vi "display_1s_stim_9s_ISI_CS1_CS2_blocks.vi"() -> ()   [LabVIEW 2019]
uses:
  <vilib>/Analysis/Matrix/Datatypes/RealMatrix.ctl
  <vilib>/Utility/file.llb/Write Delimited Spreadsheet (DBL).vi
  <vilib>/Analysis/Matrix/NI_Matrix.lvlib
panel:
  out "Active trial":bool=TRUE
  out "ISI Time":dbl
  out "Stim TS":dbl
  out "Output":dbl[][](array[numeric])
  out "Output frame":T1
  out "Frame_clock":u32
  out "Array temp1":T1
  out "Elapsed Time":dbl
  out "Display":bool=TRUE
  out "Trial":u32=1
  out "reward":dbl[](array[numeric])
  out "stim_id":dbl[](array[numeric])
  out "stim_loaded":dbl
  out "Timings":dbl[](array[numeric])
  out "Stimuli Loaded?":bool
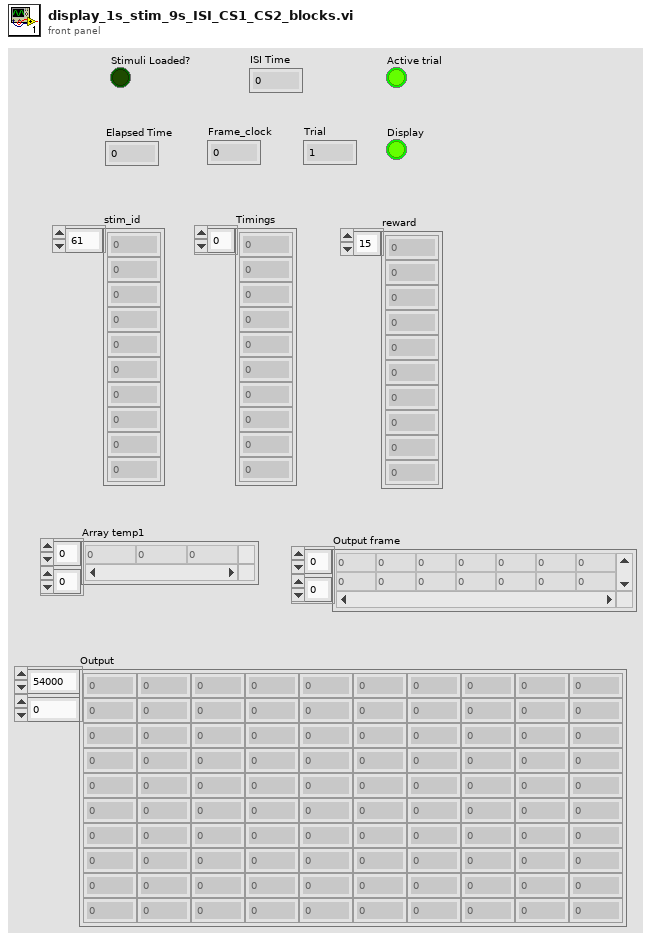
[diagram p1: front panel]
types:
  T1 = typedef "NI_Matrix.lvlib/RealMatrix.ctl" = dbl[][]
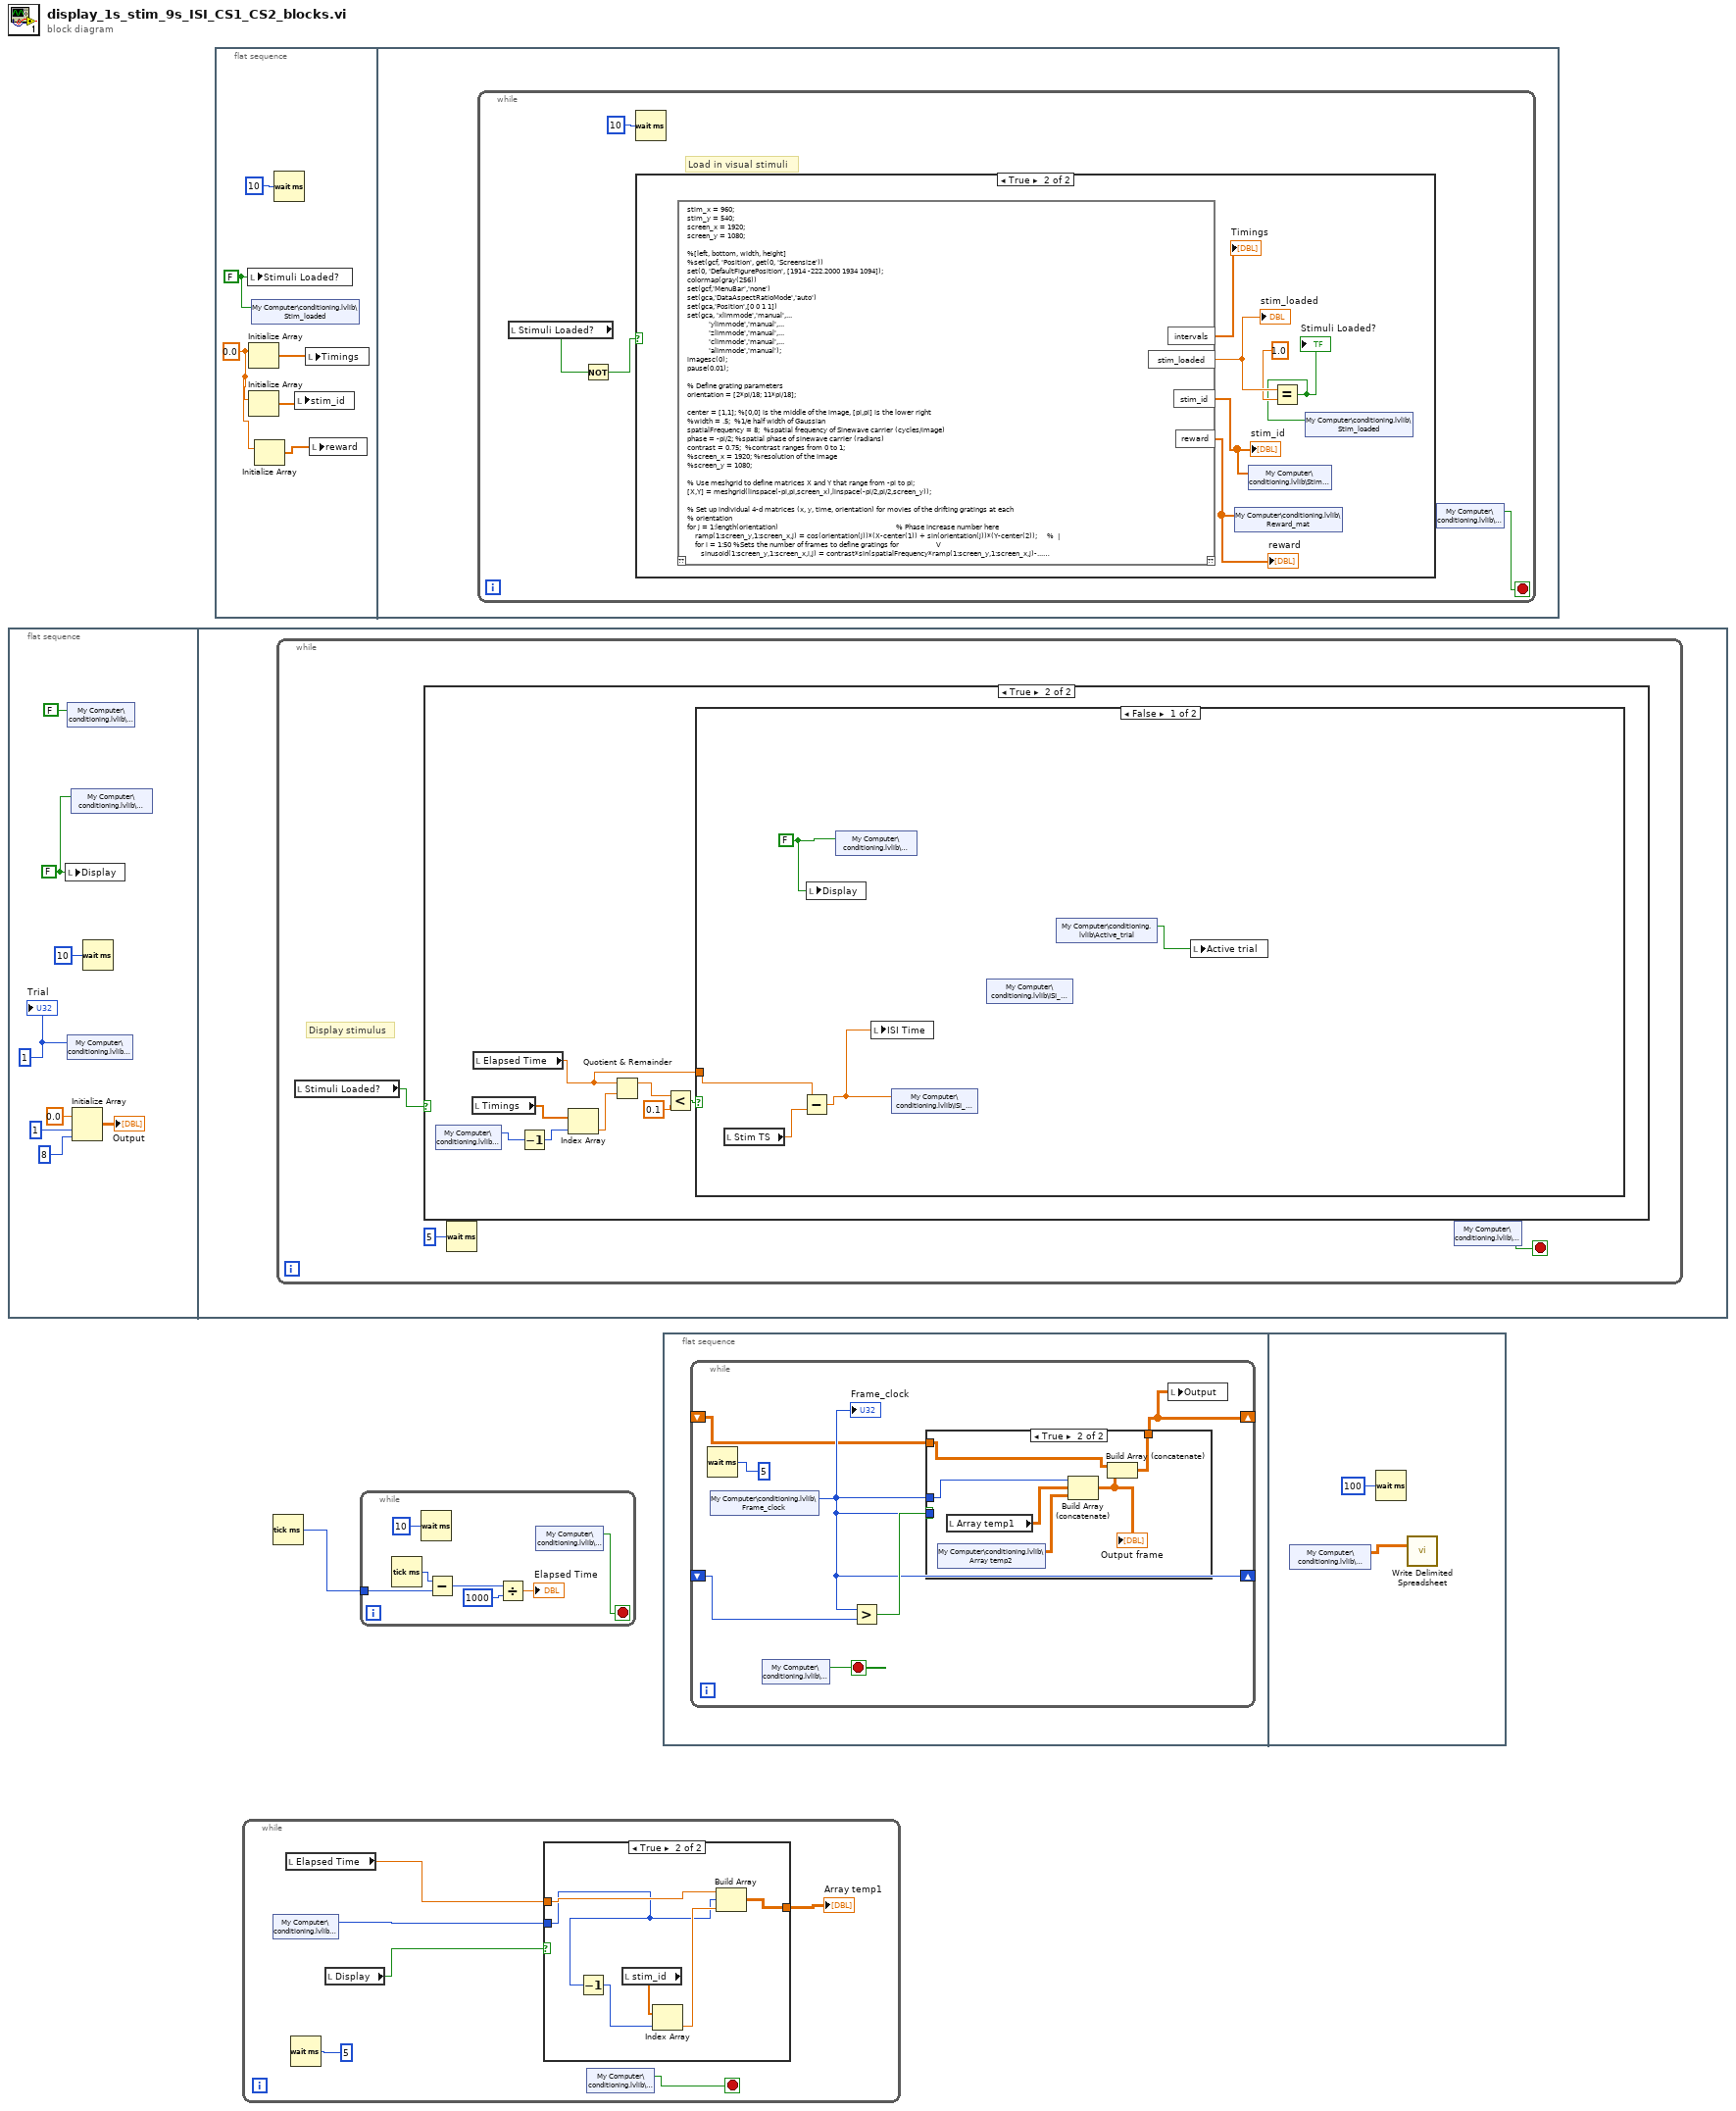
[diagram p0: block diagram]
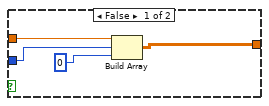
[diagram p2: hidden frame]
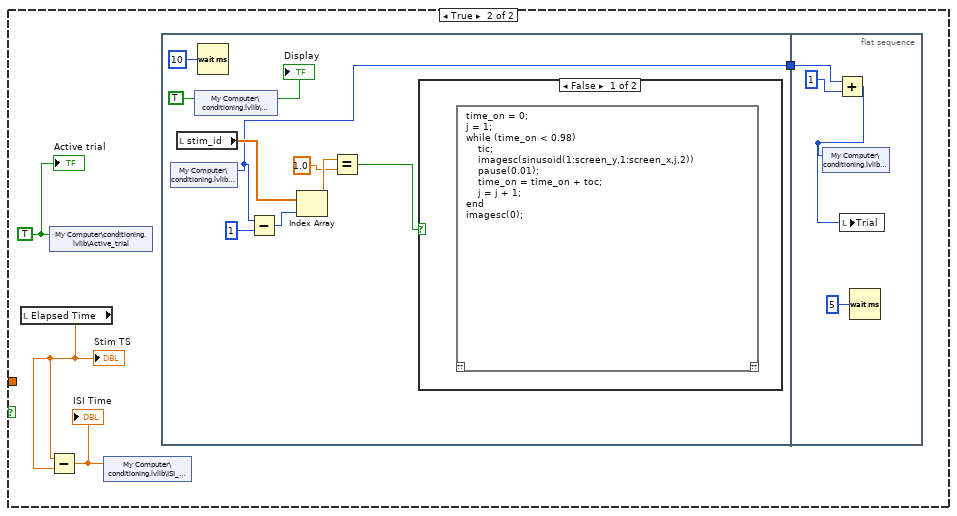
[diagram p6: hidden frame]
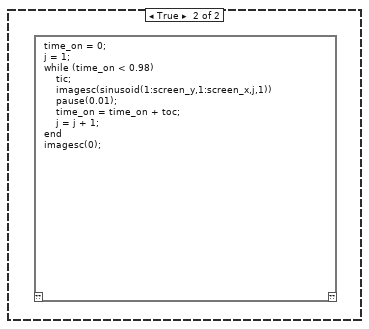
[diagram p7: hidden frame]
diagram:
  n1 = flat-sequence {
    frame #0 {
      w7 = FALSE ("Display")
      w9 = u32 1 ("Trial")
      n2 = local write "Display"(w7) -> ()
      n3 = shared-variable "My Computer\\conditioning.lvlib\\Stop"(FALSE ("Stop")) -> ()  [unwired: 1 in, 1 out]
      n4 = shared-variable "My Computer\\conditioning.lvlib\\Trial"(w9) -> ()  [unwired: 1 in, 1 out]
      n5 = shared-variable "My Computer\\conditioning.lvlib\\Display"(w7) -> ()  [unwired: 1 in, 1 out]
      n6 = Initialize Array(0.0 ("element"), 1 ("dimension size"), 8 ("dimension size")) -> (→"Output":dbl[][])
      n7 = Wait (ms)(milliseconds to wait=u32 10) -> ()  [unwired: 1 out]
      "Trial" <- w9
    }
    frame #1 {
      n8 = while {
        stop <- w11 stop-if-true
        # "Display stimulus"
        n9 = local read "Stimuli Loaded?"() -> (w10:bool)
        n10 = case shown="True" w10 {
          frame False {
          }
          frame True {
            n11 = shared-variable "My Computer\\conditioning.lvlib\\Trial"() -> (w16:u32)  [unwired: 1 in, 1 out]
            n12 = local read "Timings"() -> (w17:dbl[])
            n13 = local read "Elapsed Time"() -> (w13:dbl)
            n14 = Decrement(x=w16) -> (x-1=w15:u32)
            n15 = Index Array(array=w17, index=w15) -> (element=w14:dbl)
            n16 = Quotient & Remainder(x=w13, y=w14) -> (x-y*floor(x/y)=w20:dbl)  [unwired: 1 out]
            n17 = Less?(x=w20, y=0.1) -> (x < y?=w18:bool)
            n18 = case shown="False" w18 {
              tunnel: w13 -> [w24 _]
              frame False {
                w25 = FALSE ("Display")
                n19 = local read "Stim TS"() -> (w23:dbl)
                n20 = Subtract(x=w24, y=w23) -> (x-y=w22:dbl)
                n21 = local write "Display"(w25) -> ()
                n22 = shared-variable "My Computer\\conditioning.lvlib\\Display"(w25) -> ()  [unwired: 1 in, 1 out]
                n23 = local write "ISI Time"(w22) -> ()
                n24 = shared-variable "My Computer\\conditioning.lvlib\\ISI_Time"(w22) -> ()  [unwired: 1 in, 1 out]
                n25 = shared-variable "My Computer\\conditioning.lvlib\\ISI_Time"() -> ()  [unwired: 1 in, 2 out]
                n26 = shared-variable "My Computer\\conditioning.lvlib\\Active_trial"() -> (w21:bool)  [unwired: 1 in, 1 out]
                n27 = local write "Active trial"(w21) -> ()
              }
              frame True {
                w27 = TRUE ("Active_trial")
                n28 = local read "Elapsed Time"() -> (w28:dbl)
                "Stim TS" <- w28
                n29 = Subtract(x=w28, y=w28) -> (x-y=w26:dbl)
                "ISI Time" <- w26
                n30 = shared-variable "My Computer\\conditioning.lvlib\\Active_trial"(w27) -> ()  [unwired: 1 in, 1 out]
                n31 = shared-variable "My Computer\\conditioning.lvlib\\ISI_Time"(w26) -> ()  [unwired: 1 in, 1 out]
                n32 = flat-sequence {
                  tunnel: [w32] -> w29
                  tunnel: w29 -> [w42]
                  frame #0 {
                    w34 = TRUE ("Boolean")
                    n33 = shared-variable "My Computer\\conditioning.lvlib\\Trial"() -> (w32:u32)  [unwired: 1 in, 1 out]
                    n34 = local read "stim_id"() -> (w37:dbl[])
                    n35 = shared-variable "My Computer\\conditioning.lvlib\\Display"(w34) -> ()  [unwired: 1 in, 1 out]
                    n36 = Wait (ms)(milliseconds to wait=u32 10) -> ()  [unwired: 1 out]
                    n37 = Subtract(x=w32, y=u32 1) -> (x-y=w33:u32)
                    n38 = Index Array(array=w37, index=w33) -> (element=w36:dbl)
                    n39 = Equal?(x=w36, y=1.0) -> (x = y?=w30:bool)
                    n40 = case shown="False" w30 {
                      frame False {
                        n41 = script code="time_on = 0;\nj = 1;\nwhile (time_on < 0.98)\n    tic;\n    imagesc(sinusoid(1:screen_y,1:screen_x,j,2))\n    pause(0.01);\n    time_on = time_on + toc;\n    j = j + 1;\nend\nimagesc(0);"() -> ()  [unwired: 1 in, 1 out]
                      }
                      frame True {
                        n42 = script code="time_on = 0;\nj = 1;\nwhile (time_on < 0.98)\n    tic;\n    imagesc(sinusoid(1:screen_y,1:screen_x,j,1))\n    pause(0.01);\n    time_on = time_on + toc;\n    j = j + 1;\nend\nimagesc(0);"() -> ()  [unwired: 1 in, 1 out]
                      }
                    }
                    "Display" <- w34
                  }
                  frame #1 {
                    n43 = Add(x=w42, y=u32 1) -> (x+y=w40:u32)
                    n44 = shared-variable "My Computer\\conditioning.lvlib\\Trial"(w40) -> ()  [unwired: 1 in, 1 out]
                    n45 = local write "Trial"(w40) -> ()
                    n46 = Wait (ms)(milliseconds to wait=u32 5) -> ()  [unwired: 1 out]
                  }
                }
                "Active trial" <- w27
              }
            }
          }
        }
        n47 = Wait (ms)(milliseconds to wait=u32 5) -> ()  [unwired: 1 out]
        n48 = shared-variable "My Computer\\conditioning.lvlib\\Stop"() -> (w11:bool)  [unwired: 1 in, 1 out]
      }
    }
  }
  n49 = flat-sequence {
    frame #0 {
      w45 = 0.0 ("element")
      w43 = FALSE ("Stimuli Loaded?")
      n50 = local write "Stimuli Loaded?"(w43) -> ()
      n51 = Initialize Array(w45) -> (w47:dbl[])  [unwired: 1 in]
      n52 = Initialize Array(w45) -> (w46:dbl[])  [unwired: 1 in]
      n53 = shared-variable "My Computer\\conditioning.lvlib\\Stim_loaded"(w43) -> ()  [unwired: 1 in, 1 out]
      n54 = Initialize Array(w45) -> (w44:dbl[])  [unwired: 1 in]
      n55 = Wait (ms)(milliseconds to wait=u32 10) -> ()  [unwired: 1 out]
      n56 = local write "stim_id"(w46) -> ()
      n57 = local write "Timings"(w47) -> ()
      n58 = local write "reward"(w44) -> ()
    }
    frame #1 {
      n59 = while {
        stop <- w51 stop-if-true
        # "Load in visual stimuli"
        n60 = local read "Stimuli Loaded?"() -> (w50:bool)
        n61 = Not(x=w50) -> (.not. x?=w49:bool)
        n62 = Wait (ms)(milliseconds to wait=u32 10) -> ()  [unwired: 1 out]
        n63 = case shown="True" w49 {
          frame False {
          }
          frame True {
            n64 = script code="stim_x = 960;\nstim_y = 540;\nscreen_x = 1920;\nscreen_y = 1080;\n\n%[left, bottom, width, height]\n%set(gcf, 'Position', get(0, 'Screensize'))\nset(0, 'DefaultFigurePosition', [1914 -222.2000 1934 1094]);\ncolormap(gray(256))\nset(gcf,'MenuBar','none')\nset(gca,'DataAspectRatioMode','auto')\nset(gca,'Position',[0 0 1 1])\nset(gca, 'xlimmode','manual',...\n           'ylimmode','manual',...\n           'zlimmode','manual',...\n           'climmode','manual',...\n           'alimmode','manual');\nimagesc(0);\npause(0.01);\n\n% Define grating parameters\norientation = [2*pi/18; 11*pi/18];\n\ncenter = [1,1]; %[0,0] is the middle of the image, [pi,pi] is the lower right\n%width = .5;  %1/e half width of Gaussian\nspatialFrequency = 8;  %spatial frequency of Sinewave carrier (cycles/image)\nphase = -pi/2; %spatial phase of sinewave carrier (radians)\ncontrast = 0.75;  %contrast ranges from 0 to 1;\n%screen_x = 1920; %resolution of the image  \n%screen_y = 1080;\n\n% Use meshgrid to define matrices X and Y that range from -pi to pi;\n[X,Y] = meshgrid(linspace(-pi,pi,screen_x),linspace(-pi/2,pi/2,screen_y));\n\n% Set up individual 4-d matrices (x, y, time, orientation) for movies of the drifting gratings at each\n% orientation\nfor j = 1:length(orientation)                                                            % Phase increase number here\n    ramp(1:screen_y,1:screen_x,j) = cos(orientation(j))*(X-center(1)) + sin(orientation(j))*(Y-center(2));     %  |\n    for i = 1:50 %Sets the number of frames to define gratings for                   V\n       sinusoid(1:screen_y,1:screen_x,i,j) = contrast*sin(spatialFrequency*ramp(1:screen_y,1:screen_x,j)-...\n           (phase+(2*pi*(i-1)*(-30)/360))); %Number before '/360' sets the phase increase\n    end\nend\n\nintervals = [ones(1,204)*12];\nstim_id = [ones(1,34)*1 ones(1,34)*2 ones(1,34)*1 ones(1,34)*2 ones(1,34)*1 ones(1,34)*2];\nreward = [ones(1,204)];\n\nstim_loaded = 1;" ("Script Node")() -> ("stim_loaded"=w58:dbl, "intervals"=→"Timings":dbl[], "stim_id"=w53:dbl[], "reward"=w55:dbl[])  [unwired: 1 in, 1 out]
            "stim_loaded" <- w58
            "stim_id" <- w53
            "reward" <- w55
            n65 = shared-variable "My Computer\\conditioning.lvlib\\Reward_mat"(w55) -> ()  [unwired: 1 in, 1 out]
            n66 = shared-variable "My Computer\\conditioning.lvlib\\Stim_ID"(w53) -> ()  [unwired: 1 in, 1 out]
            n67 = Equal?(x=w58, y=1.0) -> (x = y?=w54:bool)
            "Stimuli Loaded?" <- w54
            n68 = shared-variable "My Computer\\conditioning.lvlib\\Stim_loaded"(w54) -> ()  [unwired: 1 in, 1 out]
          }
        }
        n69 = shared-variable "My Computer\\conditioning.lvlib\\Stop"() -> (w51:bool)  [unwired: 1 in, 1 out]
      }
    }
  }
  n70 = while {
    stop <- w59 stop-if-true
    n71 = shared-variable "My Computer\\conditioning.lvlib\\Trial"() -> (w61:u32)  [unwired: 1 in, 1 out]
    n72 = local read "Elapsed Time"() -> (w63:dbl)
    n73 = Wait (ms)(milliseconds to wait=u32 5) -> ()  [unwired: 1 out]
    n74 = local read "Display"() -> (w60:bool)
    n75 = case shown="True" w60 {
      tunnel: w61 -> [w67 w70]
      tunnel: w63 -> [w68 w72]
      tunnel: [w66 w73] -> w62
      frame False {
        n76 = Build Array(w68, w67, u32 0 ("milliseconds to wait")) -> (w66:T1)
      }
      frame True {
        n77 = Decrement(x=w70) -> (x-1=w69:u32)
        n78 = local read "stim_id"() -> (w74:dbl[])
        n79 = Index Array(array=w74, index=w69) -> (element=w71:dbl)
        n80 = Build Array(w72, w70, w71) -> (w73:T1)
      }
    }
    "Array temp1" <- w62
    n81 = shared-variable "My Computer\\conditioning.lvlib\\Stop"() -> (w59:bool)  [unwired: 1 in, 1 out]
  }
  n82 = Tick Count (ms)() -> (millisecond timer value=w1:u32)
  n83 = while {
    tunnel: w1 -> [w78]
    stop <- w75 stop-if-true
    n84 = Tick Count (ms)() -> (millisecond timer value=w79:u32)
    n85 = Wait (ms)(milliseconds to wait=u32 10) -> ()  [unwired: 1 out]
    n86 = Subtract(x=w79, y=w78) -> (x-y=w76:u32)
    n87 = Divide(x=w76, y=u32 1000) -> (x/y=→"Elapsed Time":dbl)
    n88 = shared-variable "My Computer\\conditioning.lvlib\\Stop"() -> (w75:bool)  [unwired: 1 in, 1 out]
  }
  n89 = flat-sequence {
    frame #0 {
      n90 = while {
        shift-right: [w84] -> _
        shift-left: _ -> [w86]
        shift-right: [w82] -> _
        shift-left: _ -> [w83]
        stop <- w88 stop-if-true
        n91 = Wait (ms)(milliseconds to wait=u32 5) -> ()  [unwired: 1 out]
        n92 = shared-variable "My Computer\\conditioning.lvlib\\Frame_clock"() -> (w84:u32)  [unwired: 1 in, 1 out]
        "Frame_clock" <- w84
        n93 = shared-variable "My Computer\\conditioning.lvlib\\Stop"() -> (w88:bool)  [unwired: 1 in, 1 out]
        n94 = Greater?(x=w84, y=w86) -> (0:w85:bool)
        n95 = case shown="True" w85 {
          tunnel: w84 -> [_ _]
          tunnel: w84 -> [_ w95]
          tunnel: [w89 w91] -> w82
          tunnel: w83 -> [w89 w90]
          frame False {
          }
          frame True {
            n96 = shared-variable "My Computer\\conditioning.lvlib\\Array temp2"() -> (w93:dbl[][])  [unwired: 1 in, 1 out]
            n97 = local read "Array temp1"() -> (w94:T1)
            n98 = Build Array (concatenate)(w95, w94, w93) -> (w92:T1)
            "Output frame" <- w92
            n99 = Build Array (concatenate) ("Build Matrix")(w90, w92) -> (w91:T1)
          }
        }
        n100 = local write "Output"(w82) -> ()
      }
    }
    frame #1 {
      n101 = shared-variable "My Computer\\conditioning.lvlib\\Output"() -> (w97:dbl[][])  [unwired: 1 in, 1 out]
      n102 = Wait (ms)(milliseconds to wait=u32 100) -> ()  [unwired: 1 out]
      n103 = call-poly <vilib>:"Write Delimited Spreadsheet.vi"("2D data"=w97) -> ()  [unwired: 13 in, 2 out]
    }
  }
